vi "CreateLogger.vi"(4 "PythonPath":path, 5 "SessionName":string, 6 "PythonVersion":string, 7 "ModulePath":path, 8 "error in (no error)":errorcluster, 11 "Name":string) -> (0 "error out":errorcluster, 3 "Logger":refnum<class "Logger.lvclass">)   [LabVIEW 2022 SP3, in "Logger.lvlib" / "Logger.lvclass"]
uses:
  Logger.lvclass
  C:/Users/jakub/repos/gh/sw4sys/lv-logger/PythonWrapper/Source/PythonSession/PythonSession.lvclass
  C:/Users/jakub/repos/gh/sw4sys/lv-logger/PythonWrapper/Source/PythonWrapper/PythonWrapper.lvclass
  C:/Users/jakub/repos/gh/sw4sys/lv-logger/Logger/Source/LoggingWrapper/LoggingWrapper.lvclass
  PythonWrapper/Source/PythonSession/PythonSession.lvclass/PythonSession.ctl
  PythonWrapper/Source/PythonWrapper/PythonWrapper.lvclass/PythonWrapper.ctl
  LoggingWrapper/LoggingWrapper.lvclass/LoggingWrapper.ctl
  Logger.lvclass/Logger.ctl
  PythonWrapper/Source/PythonSession/Write SessionName.vi
  PythonWrapper/Source/PythonSession/Write PythonVersion.vi
  PythonWrapper/Source/PythonSession/Write PythonPath.vi
  PythonWrapper/Source/PythonWrapper/Write ModulePath.vi
  PythonWrapper/Source/PythonSession/Read PythonSession.vi
  PythonWrapper/Source/PythonWrapper/Read ModulePath.vi
  Write Name.vi
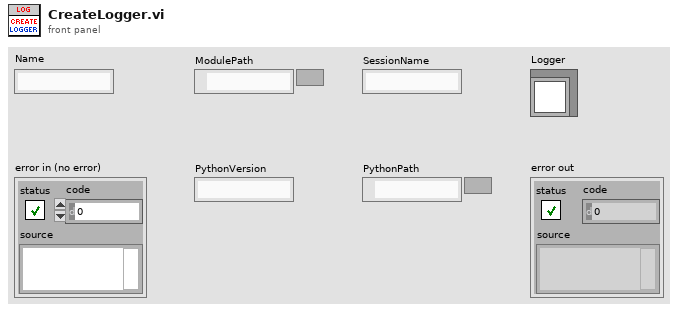
[diagram p1: front panel]
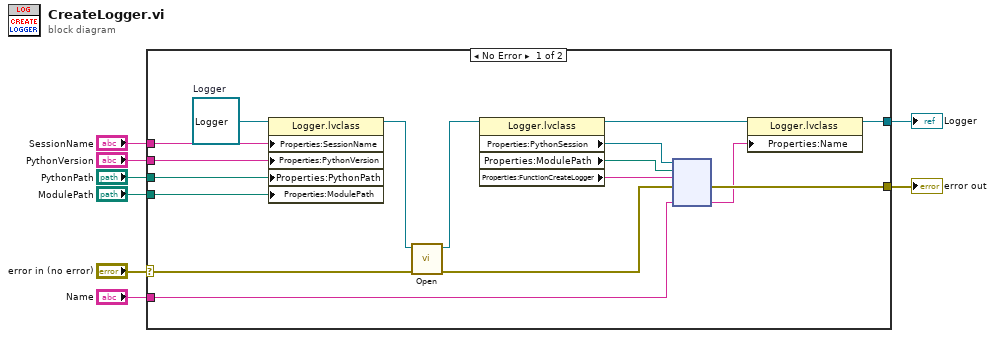
[diagram p0: block diagram]
diagram:
  n1 = case shown="No Error" "error in (no error)" {
    selector: "error in (no error)" -> [w17 w26]
    tunnel: [w20 w26] -> w7
    tunnel: [w21 _] -> w6
    tunnel: "Name" -> [w15 _]
    tunnel: "ModulePath" -> [w12 _]
    tunnel: "PythonVersion" -> [w14 _]
    tunnel: "PythonPath" -> [w13 _]
    tunnel: "SessionName" -> [w9 _]
    frame No Error {
      w18 = refnum<class "Logger.lvclass"> refnum  # Logger
      n2 = property class="Logger.lvclass"(reference=w18, "Properties:SessionName"=w9, "Properties:PythonVersion"=w14, "Properties:PythonPath"=w13, "Properties:ModulePath"=w12) -> (reference out=w11:refnum<class "Logger.lvclass">)  [unwired: 1 in, 1 out]
      n3 = call-dynamic "Open.vi"("error in (no error)"=w17, "PythonWrapper in"=w11) -> ("error out"=w16:errorcluster, "PythonWrapper out"=w10:refnum<class "Logger.lvclass">)  [unwired: 8 in]
      n4 = property class="Logger.lvclass"(reference=w10) -> (reference out=w22:refnum<class "Logger.lvclass">, "Properties:PythonSession"=w25:refnum<k35>, "Properties:ModulePath"=w24:path, "Properties:FunctionCreateLogger"=w23:string)  [unwired: 1 in, 1 out]
      n5 = node(w25, w24, w23, w16, w15) -> (w20:errorcluster, w19:string)  [unwired: 2 in, 3 out]
      n6 = property class="Logger.lvclass"(reference=w22, "Properties:Name"=w19) -> (reference out=w21:refnum<class "Logger.lvclass">)  [unwired: 1 in, 1 out]
    }
    frame Error {
    }
  }
  "error out" <- w7
  "Logger" <- w6
